vi "Read List of Worksheets.vi"(8 "error in (no error)":errorcluster, 11 "Excel Saver in":refnum<class "Excel Saver.lvclass">) -> (0 "error out":errorcluster, 2 "List of Worksheets":string[](array[string]), 3 "Excel Saver out":refnum<class "Excel Saver.lvclass">)   [LabVIEW 2016, in "Data Saving.lvlib" / "Excel Saver.lvclass"]
uses:
  Excel Saver.lvclass
  Excel Saver.lvclass/Excel Saver.ctl
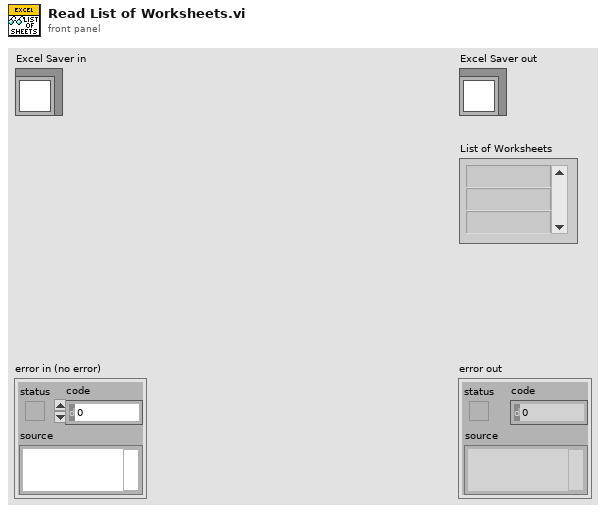
[diagram p1: front panel]
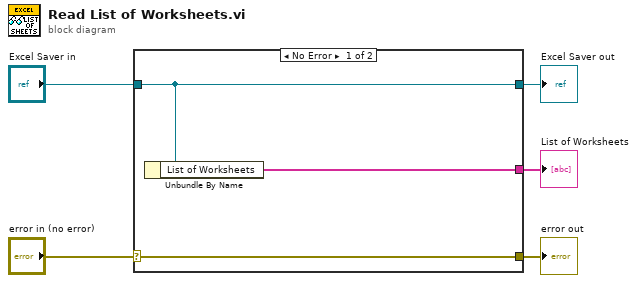
[diagram p0: block diagram]
diagram:
  n1 = case shown="No Error" "error in (no error)" {
    selector: "error in (no error)" -> [w8 w9]
    tunnel: [w8 w9] -> w4
    tunnel: [w7 w10] -> w2
    tunnel: "Excel Saver in" -> [w7 w10]
    tunnel: [w6 _] -> w1
    frame No Error {
      n2 = Unbundle By Name(w7) -> ("List of Worksheets"=w6:string[])
    }
    frame Error {
    }
  }
  "error out" <- w4
  "Excel Saver out" <- w2
  "List of Worksheets" <- w1
